vi "crdDisplayFit_poly.vi"   [LabVIEW 2011]
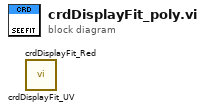
[diagram p0: block diagram]
diagram:
  n1 = call "crdDisplayFit_UV.vi"() -> ()  [unwired: 11 in, 1 out]
  n2 = call "crdDisplayFit_Red.vi"() -> ()  [unwired: 11 in, 1 out]
